vi "CreateBall.vi"(8 "error in (no error)":errorcluster, 10 "velocity in":sgl, 11 "class data in":refnum<class "Ball.lvclass">) -> (0 "error out":errorcluster, 3 "class data out":refnum<class "Ball.lvclass">)   [LabVIEW 2010, in "Labricks.lvlib" / "Ball.lvclass"]
uses:
  Ball.lvclass
  RenderBase/SceneObject_class/SceneObject.lvclass
  Ball.lvclass/Ball.ctl
  <vilib>/picture/3D Picture Control/NI_3D Picture Control.lvlib
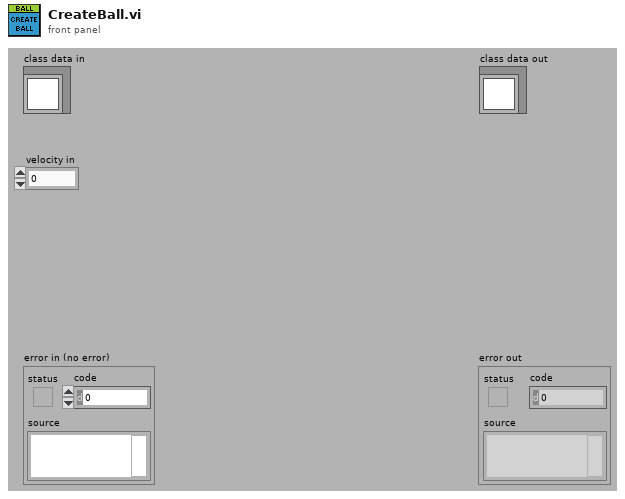
[diagram p1: front panel]
types:
  T1 = cluster{"Red":sgl, "Green":sgl, "Blue":sgl, "Alpha":sgl}
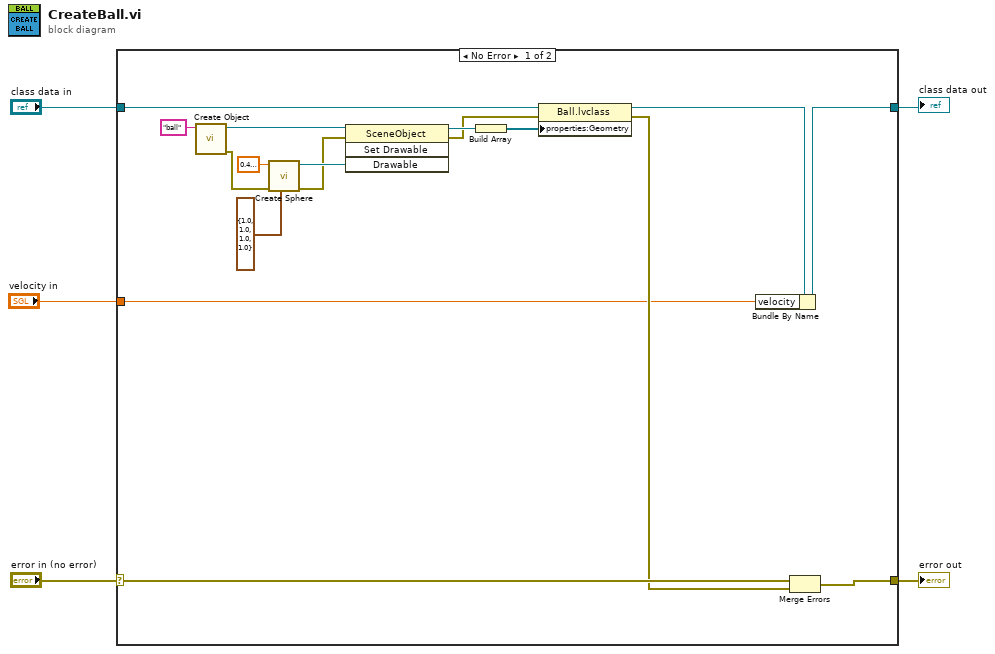
[diagram p0: block diagram]
diagram:
  n1 = case shown="No Error" "error in (no error)" {
    selector: "error in (no error)" -> [w22 w24]
    tunnel: [w10 w24] -> w4
    tunnel: "class data in" -> [w21 w23]
    tunnel: [w7 w23] -> w2
    tunnel: "velocity in" -> [w6 _]
    frame No Error {
      n2 = call <vilib>:"Create Object.vi"("Name"="ball") -> ("error out"=w13:errorcluster, "Scene:New Object"=w18:refnum<vi>)  [unwired: 9 in]
      n3 = call <vilib>:"Create Sphere.vi"("Color"=T1 {"Red"=1.0, "Green"=1.0, "Blue"=1.0, "Alpha"=1.0}, "error in (no error)"=w13, "Radius"=sgl 0.4) -> ("error out"=w12:errorcluster, "New Sphere Refnum"=w20:refnum<vi>)  [unwired: 7 in]
      n4 = invoke class="SceneObject" method="Set Drawable"(reference=w18, error in=w12, "Drawable"=w20) -> (reference out=w17:refnum<vi>, error out=w11:errorcluster)  [unwired: 1 in, 2 out]
      n5 = Build Array(w17) -> (w14:refnum<vi>[])
      n6 = property class="Ball.lvclass"(reference=w21, error in=w11, "properties:Geometry"=w14) -> (reference out=w8:refnum<class "Ball.lvclass">, error out=w9:errorcluster)
      n7 = Bundle By Name(cluster=w8, "velocity"=w6) -> (w7:refnum<class "Ball.lvclass">)
      n8 = Merge Errors(w22, w9) -> (w10:errorcluster)
    }
    frame Error {
    }
  }
  "error out" <- w4
  "class data out" <- w2
